vi "PV HLT5xx Calibration.vi"(0 "VISA session":refnum<visa-resource-name>, 1 "Adress of unit":u16=1 min=1 max=999 step=1, 5 "Parameter":u16(ring) items=[" Calibration State", " Acknowledge calibrationsteps", " Leakrate external testleak vacuum", " Leakrate external testleak sniff", " Leakrate internal testleak", " Calibration factor high (read only)", " Calibration factor low (read only)", " Calibration factor counter flow (read only) "], 7 "Parameter\nread only<->describe":bool, 9 "Acknowledge\nCalibrationsteps":u16(ring)=1 items=["Cancel", "ok"], 11 "error in (no error)":errorcluster, 12 "Leakrate value in":dbl=1e-07 format="%.2e") -> (4 "dup VISA session":refnum<visa-resource-name>, 6 "response (data)":string, 10 "Calibration state out":i8(ring) items=["--", "Connect TL", "Pumping", "Measure TF high", "Massadjust", "Calibrate TF high", "Calibrate TF low", "Calibrate Counter Flow", "Remove TL", "Background TF high", "Background TF low", "Background Counter Flow", "Wait for confirmation"], 15 "error out":errorcluster)   [LabVIEW 2016, in "Pfeiffer Vacuum.lvlib"]
doc: "There are 8 parameters available, only one of which can be enabled at a time. \n\n0 - Calibration State (default) - Para 667\n1 - Acknowledge calibrationsteps - Para 668\n2 - Leakrate external testleak vacuum - Para 671\n3 - Leakrate external testleak sniff - Para 673\n4 - Leakrate internal testleak - Para 676\n5 - Calibration factor high (read only) - Para 694\n6 - Calibration factor low (read only) - Para 695\n7 - Calibration factor counter flow (read only) - Para 696\n\nNote: The 3 controls down of this one will set the appropriate values for the selected parameter. Any settings for an parameter that is not selected will be ignored. If a value is out of range, it will be changed to either the upper or the lower limit of the range."
uses:
  Pfeiffer Vacuum.lvlib
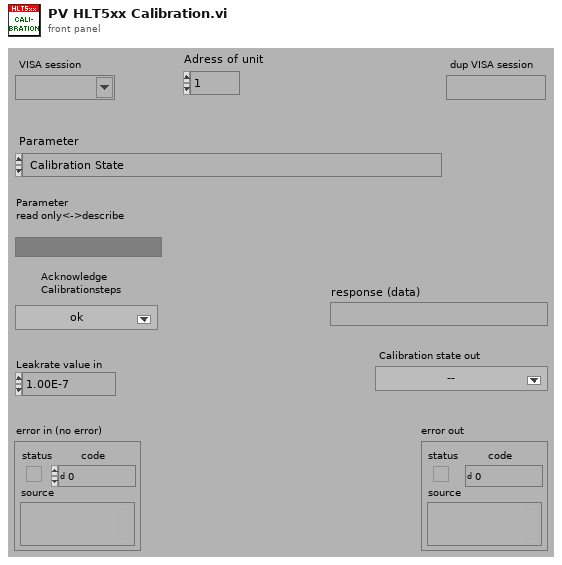
[diagram p1: front panel]
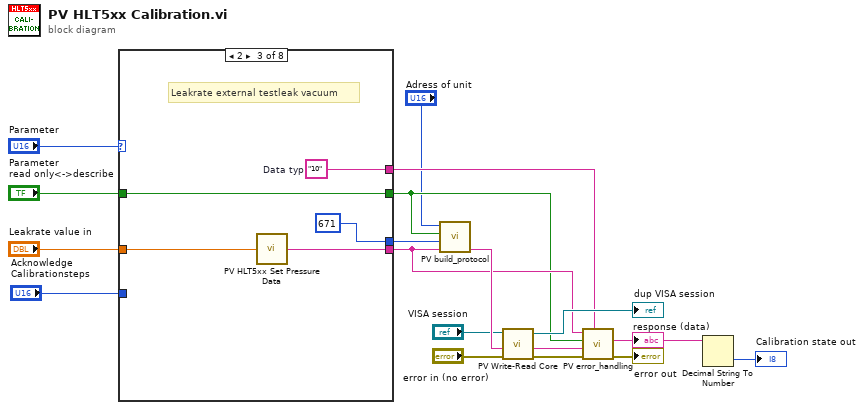
[diagram p0: block diagram]
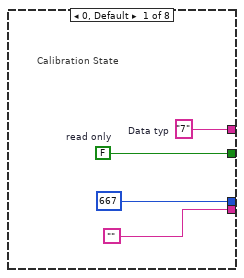
[diagram p2: hidden frame]
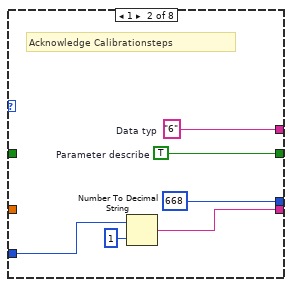
[diagram p3: hidden frame]
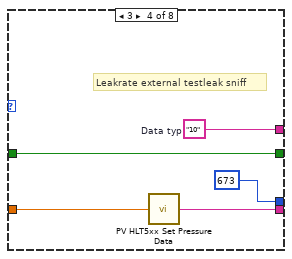
[diagram p4: hidden frame]
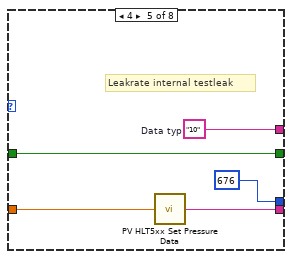
[diagram p5: hidden frame]
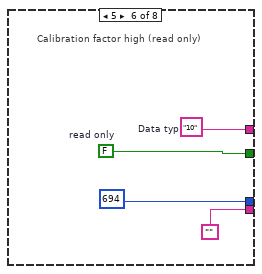
[diagram p6: hidden frame]
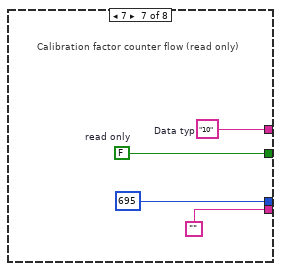
[diagram p7: hidden frame]
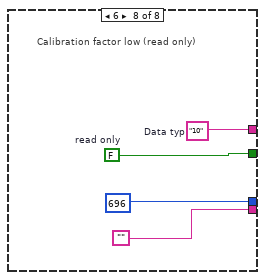
[diagram p8: hidden frame]
diagram:
  n1 = case shown="2" "Parameter" {
    tunnel: [u16 667 ("Parameter-number") u16 668 ("Parameter-number") u16 671 ("Parameter-number") u16 673 ("Parameter-number") u16 676 ("Parameter-number") u16 694 ("Parameter-number") u16 695 ("Parameter-number") u16 696 ("Parameter-number")] -> w18
    tunnel: ["" w24 w29 w35 w39 "" "" ""] -> w13
    tunnel: [w21 w26 w31 w37 w42 w46 w50 w55] -> w11
    tunnel: "Parameter\nread only<->describe" -> [_ _ w31 w37 w42 _ _ _]
    tunnel: [w22 w27 w33 w38 w43 w47 w51 w54] -> w12
    tunnel: "Leakrate value in" -> [_ _ w30 w34 w40 _ _ _]
    tunnel: "Acknowledge\nCalibrationsteps" -> [_ w23 _ _ _ _ _ _]
    frame 0, Default {
      w21 = FALSE  # read only
      w22 = "7"  # Data typ
      # "Calibration State"
    }
    frame 1 {
      w26 = TRUE  # Parameter describe
      w27 = "6"  # Data typ
      # "Acknowledge Calibrationsteps"
      n2 = Number To Decimal String(number=w23, width (-)=i16 1 ("Breite (-)")) -> (decimal integer string=w24:string)
    }
    frame 2 {
      w33 = "10"  # Data typ
      # "Leakrate external testleak vacuum"
      n3 = call "PV HLT5xx Set Pressure Data.vi"("Value in"=w30) -> ("Output"=w29:string)
    }
    frame 3 {
      w38 = "10"  # Data typ
      # "Leakrate external testleak sniff"
      n4 = call "PV HLT5xx Set Pressure Data.vi"("Value in"=w34) -> ("Output"=w35:string)
    }
    frame 4 {
      w43 = "10"  # Data typ
      # "Leakrate internal testleak"
      n5 = call "PV HLT5xx Set Pressure Data.vi"("Value in"=w40) -> ("Output"=w39:string)
    }
    frame 5 {
      w46 = FALSE  # read only
      w47 = "10"  # Data typ
      # "Calibration factor high (read only)"
    }
    frame 7 {
      w50 = FALSE  # read only
      w51 = "10"  # Data typ
      # "Calibration factor counter flow (read only)"
    }
    frame 6 {
      w55 = FALSE  # read only
      w54 = "10"  # Data typ
      # "Calibration factor low (read only)"
    }
  }
  n6 = call "PV build_protocol.vi"("Data"=w13, "Parameter-number"=w18, "parameter\nread<->describe"=w11, "Adress"="Adress of unit") -> ("output"=w17:string)  [unwired: 3 in]
  n7 = call "PV Write-Read Core.vi"("error in"="error in (no error)", "Write data in"=w17, "VISA session"="VISA session") -> ("error out"=w15:errorcluster, "response (data) out"=w16:string, "dup VISA session"=→"dup VISA session":refnum<visa-resource-name>)  [unwired: 2 in]
  n8 = call "PV error_handling.vi"("Data Typ in"=w12, "error in"=w15, "response (data) in"=w16, "Parameter\nread only<->describe"=w11, "data in"=w13) -> ("error out"=→"error out":errorcluster, "Data out"=w9:string)  [unwired: 4 in, 1 out]
  "response (data)" <- w9
  n9 = Decimal String To Number(string=w9) -> (number=→"Calibration state out":i32)  [unwired: 2 in, 1 out]
